vi "GenerateFilePaths.vi"() -> ()   [LabVIEW 2012]
uses:
  AppPaths.ctl
  PathTraveler.ctl
  PathTypes.ctl
panel:
  in  "AppPaths":refnum<vi>
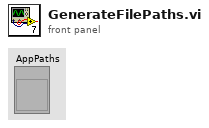
[diagram p1: front panel]
types:
  T1 = typedef "AppPaths.ctl" = cluster{"DataDir":T2, "OmniDriver":T2, "OmniDriverCommon":T2, "Configuration":T2, "WaferImage":T2}
  T2 = typedef "PathTraveler.ctl" = cluster{"Enum":T3, "FileName":string, "Exists?":bool, "Path":path}
  T3 = typedef "PathTypes.ctl" = enum16{"DataDir", "OmniDriver", "OmniDriver_Common", "Configuration", "WaferImage"}
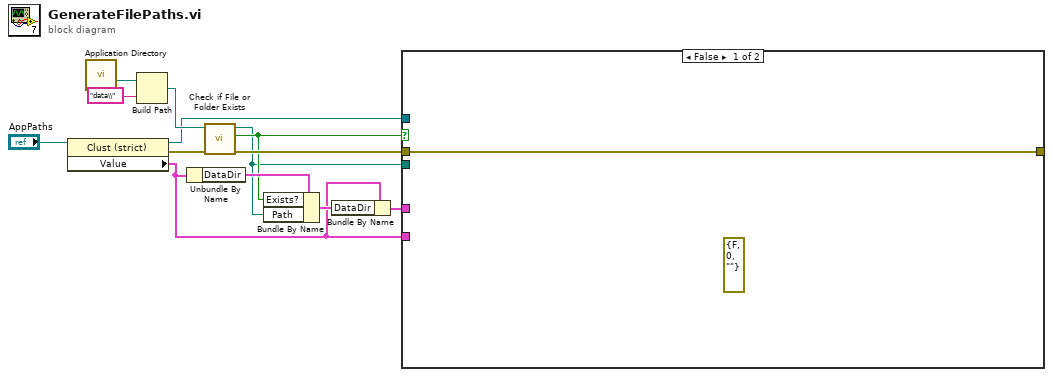
[diagram p0: block diagram]
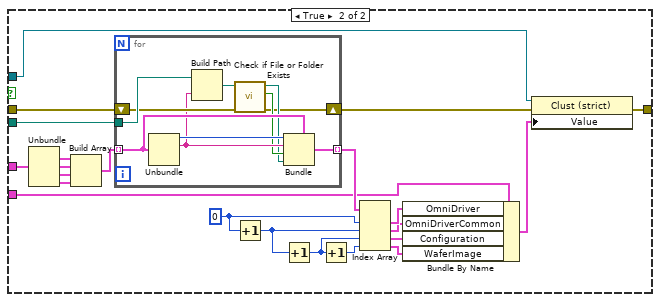
[diagram p2: hidden frame]
diagram:
  n1 = property class="Clust (strict)"(reference="AppPaths") -> (reference out=w1:refnum<vi>, error out=w2:errorcluster, "Value"=w3:T1)  [unwired: 1 in]
  n2 = call <vilib>:"Application Directory.vi"() -> ("Application Directory"=w12:path)
  n3 = Build Path(base path=w12, name or relative path="data\\") -> (appended path=w10:path)
  n4 = Unbundle By Name(w3) -> ("DataDir"=w8:T2)
  n5 = call <vilib>:"Check if File or Folder Exists.vi"("error in (no error)"=w2, "path"=w10) -> ("error out"=w9:errorcluster, "file or folder exists?"=w5:bool, "dup path"=w4:path)  [unwired: 7 in]
  n6 = Bundle By Name(cluster=w8, "Exists?"=w5, "Path"=w4) -> (w7:T2)
  n7 = Bundle By Name(cluster=w3, "DataDir"=w7) -> (w6:T1)
  n8 = case shown="False" w5 {
    tunnel: w9 -> [w14 w29]
    tunnel: w6 -> [_ w36]
    tunnel: w4 -> [_ w30]
    tunnel: w3 -> [_ w19]
    tunnel: w1 -> [_ w18]
    tunnel: [w14 w15] -> _
    frame False {
      (unwired) errorcluster {"status"=FALSE, "code"=0, "source"=""} ("error in (no error)")
    }
    frame True {
      w27 = 0 ("index")
      n9 = Unbundle(w36) -> ("OmniDriver"=w35:T2, "OmniDriverCommon"=w34:T2, "Configuration"=w33:T2, "WaferImage"=w32:T2)  [unwired: 1 out]
      n10 = Build Array(w35, w34, w33, w32) -> (w31:T2[])
      n11 = for {
        tunnel: w31 -> [w43] mode=indexing
        tunnel: w30 -> [w45]
        tunnel: [w42] -> w28 mode=indexing
        shift-right: [w37] -> w16
        shift-left: w29 -> [w44]
        n12 = Unbundle(w43) -> ("Enum"=w41:T3, "FileName"=w40:string)  [unwired: 2 out]
        n13 = Build Path(base path=w45, name or relative path=w40) -> (appended path=w46:path)
        n14 = call <vilib>:"Check if File or Folder Exists.vi"("error in (no error)"=w44, "path"=w46) -> ("error out"=w37:errorcluster, "file or folder exists?"=w39:bool, "dup path"=w38:path)  [unwired: 7 in]
        n15 = Bundle(cluster=w43, "Enum"=w41, "FileName"=w40, "Exists?"=w39, "Path"=w38) -> (w42:T2)
      }
      n16 = Increment(x=w27) -> (x+1=w26:i32)
      n17 = Increment(x=w26) -> (x+1=w24:i32)
      n18 = Increment(x=w24) -> (x+1=w25:i32)
      n19 = Index Array(array=w28, index #1=w27, index #2=w26, index #3=w24, index #4=w25) -> (element #1=w23:T2, element #2=w22:T2, element #3=w21:T2, element #4=w20:T2)
      n20 = Bundle By Name(cluster=w19, "OmniDriver"=w23, "OmniDriverCommon"=w22, "Configuration"=w21, "WaferImage"=w20) -> (w17:T1)
      n21 = property class="Clust (strict)"(reference=w18, error in=w16, "Value"=w17) -> (error out=w15:errorcluster)  [unwired: 1 out]
    }
  }
